vi "Ephys Control.vi"(11 "Trial In Progress IN":T1) -> (2 "ephys_clock freq (hz)":dbl, 3 "Boolean":bool)   [LabVIEW 2018]
uses:
  controls/Trial Config Settings.ctl
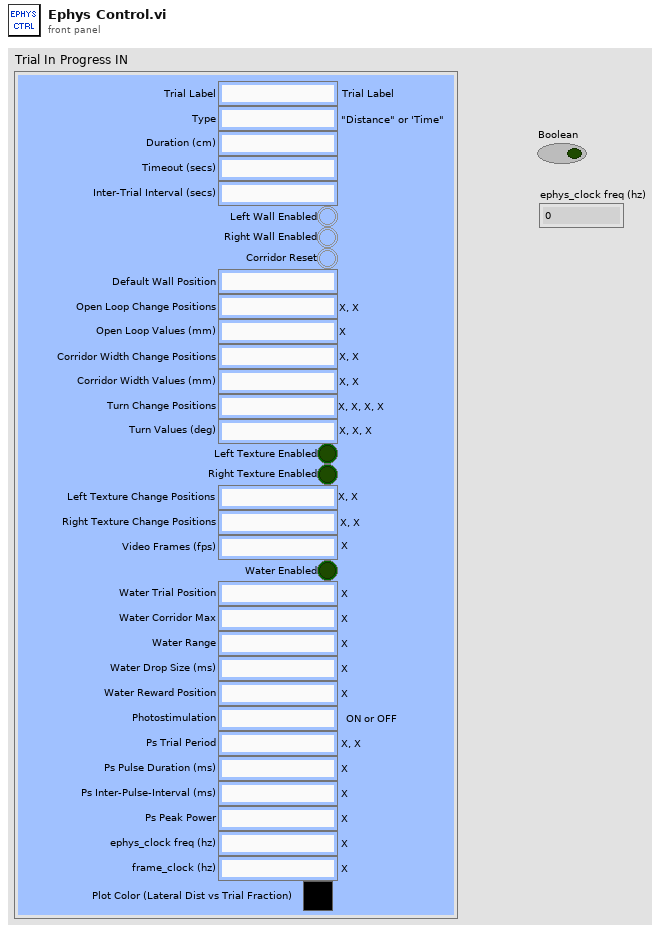
[diagram p1: front panel]
types:
  T1 = typedef "Trial Config Settings.ctl" = cluster{"Trial Label":string, "Type":string, "Timeout (secs)":string, "Inter-Trial Interval (secs)":string, "Left Wall Enabled":bool, "Right Wall Enabled":bool, "Corridor Reset":bool, "Default Wall Position":string, "Open Loop Change Positions":string, "Open Loop Values (mm)":string, "Corridor Width Change Positions":string, "Corridor Width Values (mm) ":string, "Turn Change Positions":string, "Turn Values (deg)":string, "Left Texture Change Positions":string, "Right Texture Change Positions":string, "Video Frames (fps)":string, "Water Enabled":bool, "Water Trial Position":string, "Photostimulation":string, "Water Corridor Max":string, "Water Range":string, "Water Drop Size (ms)":string, "Water Reward Position":string, "Duration (cm)":string, "Left Texture Enabled":bool, "Right Texture Enabled":bool, "Ps Trial Period":string, "Ps Inter-Pulse-Interval (ms)":string, "Ps Peak Power":string, "Ps Pulse Duration (ms)":string, "ephys_clock freq (hz)":string, "frame_clock (hz)":string, "Plot Color (Lateral Dist vs Trial Fraction)":u32}
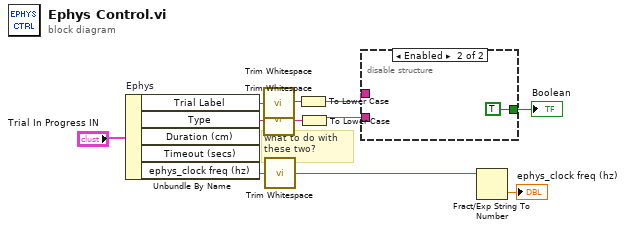
[diagram p0: block diagram]
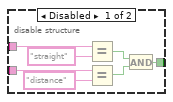
[diagram p2: hidden frame]
diagram:
  # "what to do with these two?"
  n1 = Unbundle By Name "Ephys"("Trial In Progress IN") -> ("Trial Label"=w7:string, "Type"=w9:string, "ephys_clock freq (hz)"=w3:string)  [unwired: 2 out]
  n2 = call <vilib>:"Trim Whitespace.vi"("string"=w7) -> ("trimmed string"=w8:string)  [unwired: 1 in]
  n3 = call <vilib>:"Trim Whitespace.vi"("string"=w9) -> ("trimmed string"=w10:string)  [unwired: 1 in]
  n4 = call <vilib>:"Trim Whitespace.vi"("string"=w3) -> ("trimmed string"=w2:string)  [unwired: 1 in]
  n5 = To Lower Case(string=w8) -> (all lower case string=w4:string)
  n6 = To Lower Case(string=w10) -> (all lower case string=w5:string)
  n7 = disable-structure shown="Enabled" {
    disable-tunnel: [w18 TRUE ("Boolean")] -> w6
    disable-tunnel: w5 -> [w17 _]
    disable-tunnel: w4 -> [w16 _]
    frame Disabled {
      n8 = Equal?(x=w16, y="straight") -> (x = y?=w14:bool)
      n9 = Equal?(x=w17, y="distance") -> (x = y?=w15:bool)
      n10 = And(x=w14, y=w15) -> (x .and. y?=w18:bool)
    }
    frame Enabled {
    }
  }
  "Boolean" <- w6
  n11 = Fract/Exp String To Number(string=w2) -> (number=→"ephys_clock freq (hz)":dbl)  [unwired: 3 in, 1 out]
